vi "Write Devices.vi"(10 "Devices":refnum<class "Device.lvclass">[](array[class]), 11 "Test Framework in":refnum<class "Test Framework.lvclass">) -> (3 "Test Framework out":refnum<class "Test Framework.lvclass">)   [LabVIEW 2020, in "Test Framework.lvclass"]
uses:
  Test Framework.lvclass
  Devices/Device.lvclass
  Test Framework.lvclass/Test Framework.ctl
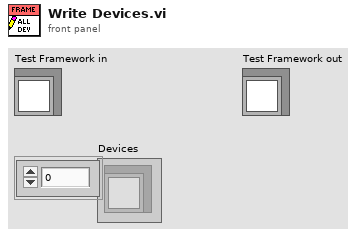
[diagram p1: front panel]
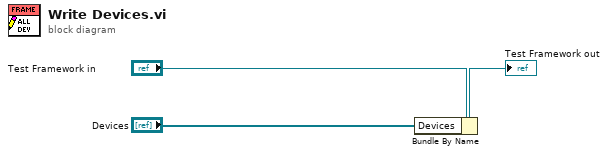
[diagram p0: block diagram]
diagram:
  n1 = Bundle By Name(cluster="Test Framework in", "Devices"="Devices") -> (→"Test Framework out":refnum<class "Test Framework.lvclass">)
